vi "get_path_wget.vi"(8 "error in (no error)":errorcluster) -> (0 "error out":errorcluster, 3 "wget":path)   [LabVIEW 2015, in "lv-bin-wget.lvlib"]
uses:
  lv-bin-wget.lvlib
  public/_controls/error.ctl
  <userlib>/antonio-alexander/lv-bin/lv-bin/public/api/v1/v1.lvlib
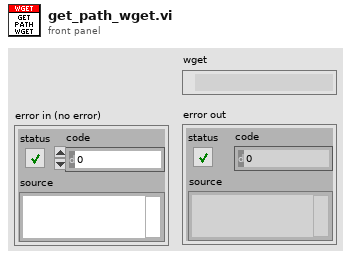
[diagram p1: front panel]
types:
  T1 = typedef "lv-bin-wget.lvlib/error.ctl" = enum16{"<error>", "wget_x86_missing", "wget_x64_missing"}
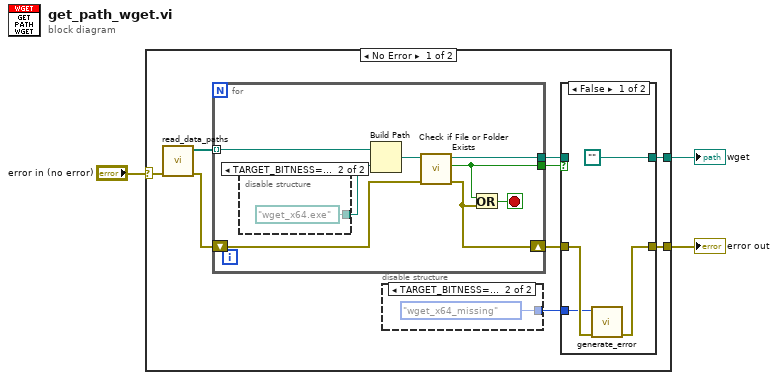
[diagram p0: block diagram]
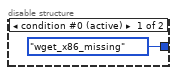
[diagram p2: hidden frame]
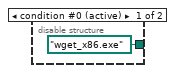
[diagram p4: hidden frame]
diagram:
  n1 = case shown="No Error" "error in (no error)" {
    selector: "error in (no error)" -> [w12 w31]
    tunnel: [w5 w31] -> w3
    tunnel: [w7 _] -> w1
    frame No Error {
      n2 = call <userlib>:"read_data_paths.vi"("error in (no error)"=w12) -> ("error out"=w11:errorcluster, "path [] out"=w10:path[])  [unwired: 9 in]
      n3 = for {
        tunnel: w10 -> [w26] mode=indexing
        shift-right: [w25] -> w6
        shift-left: w11 -> [w28]
        tunnel: [w27] -> w9
        tunnel: [w23] -> w8
        stop <- w24 stop-if-true
        n4 = disable-structure shown="TARGET_BITNESS==64" {
          disable-tunnel: [path "wget_x86.exe" ("Application Directory") path "wget_x64.exe" ("Application Directory")] -> w21
          frame condition #0 (active) {
          }
          frame condition #1 {
          }
        }
        n5 = Build Path(base path=w26, name or relative path=w21) -> (appended path=w22:path)
        n6 = call <vilib>:"Check if File or Folder Exists.vi"("error in (no error)"=w28, "path"=w22) -> ("error out"=w25:errorcluster, "file or folder exists?"=w23:bool, "dup path"=w27:path)  [unwired: 7 in]
        n7 = Or(x=w23, y=w25) -> (x .or. y?=w24:bool)
      }
      n8 = disable-structure shown="TARGET_BITNESS==64" {
        disable-tunnel: [error."wget_x86_missing" ("error") error."wget_x64_missing" ("error")] -> w4
        frame condition #0 (active) {
        }
        frame condition #1 {
        }
      }
      n9 = case shown="False" w8 {
        tunnel: w9 -> [_ w20]
        tunnel: [path "" w20] -> w7
        tunnel: w6 -> [w17 w19]
        tunnel: [w16 w19] -> w5
        tunnel: w4 -> [w15 _]
        frame False {
          n10 = call "generate_error.vi"("error in (no error)"=w17, "error"=w15) -> ("error out"=w16:errorcluster)  [unwired: 9 in]
        }
        frame True {
        }
      }
    }
    frame Error {
    }
  }
  "error out" <- w3
  "wget" <- w1
